vi "Parse Controls for xVDTs.vi"(2 "error in (no error)":errorcluster, 3 "Control Scalars":T2) -> (0 "error out":errorcluster, 1 "xVDTs":T1[](array[typedef]))   [LabVIEW 2011, in "Sensor Simulation Custom Device.lvlib"]
uses:
  Sensor Simulation Custom Device.lvlib
  <userlib>/_FPGA Interface Advanced Tools/FPGA Bitfile Utility/TypeDefs/Scalar Register Set.ctl
  <userlib>/_FPGA Interface Advanced Tools/FPGA Bitfile Utility/TypeDefs/Scalar Register.ctl
  TypeDefs/xVDT.ctl
  <vilib>/regexp/Match Regular Expression.xnode
  <userlib>/_FPGA Interface Advanced Tools/FPGA Bitfile Utility/FPGA Bitfile Utility.lvlib
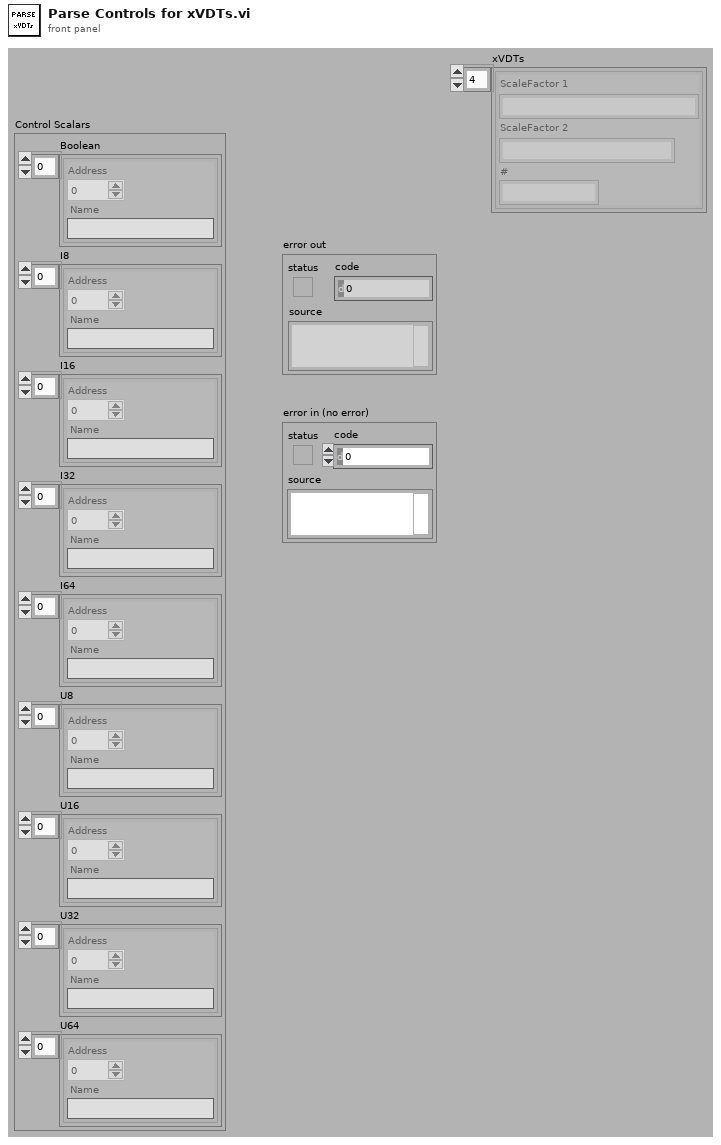
[diagram p1: front panel]
types:
  T1 = typedef "Sensor Simulation Custom Device.lvlib/xVDT.ctl" = cluster{"ScaleFactor 1":string, "ScaleFactor 2":string, "#":string}
  T2 = typedef "FPGA Bitfile Utility.lvlib/Scalar Register Set.ctl" = cluster{"Boolean":T3[], "I8":T3[], "I16":T3[], "I32":T3[], "I64":T3[], "U8":T3[], "U16":T3[], "U32":T3[], "U64":T3[]}
  T3 = typedef "FPGA Bitfile Utility.lvlib/Scalar Register.ctl" = cluster{"Address":u32, "Name":string}
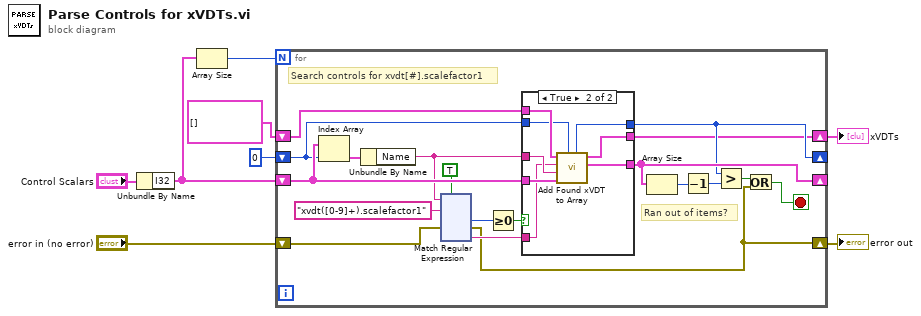
[diagram p0: block diagram]
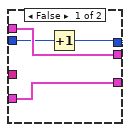
[diagram p2: hidden frame]
diagram:
  n1 = Unbundle By Name("Control Scalars") -> ("I32"=w3:T3[])
  n2 = Array Size(array=w3) -> (size(s)=w8:i32)
  n3 = for {
    N: w8 -> [_]
    shift-right: [w18] -> w4
    shift-left: T1[] [] -> [w26]
    shift-right: [w23] -> _
    shift-left: w3 -> [w25]
    shift-right: [w22] -> _
    shift-left: 0 -> [w17]
    shift-right: [w9] -> w1
    shift-left: "error in (no error)" -> [w11]
    stop <- w10 stop-if-true
    # "Search controls for xvdt[#].scalefactor1"
    # "Ran out of items?"
    n4 = Index Array(array=w25, index=w17) -> (element=w24:T3)
    n5 = Unbundle By Name(w24) -> ("Name"=w16:string)
    n6 = xnode "Match Regular Expression"("input string"=w16, "regular expression"="xvdt([0-9]+).scalefactor1", "error in"=w11, "ignore case? (F)"=TRUE) -> ("offset past match"=w13:i32, "error out"=w9:errorcluster, "submatch 1"=w12:string)  [unwired: 2 in, 3 out]
    n7 = Greater Or Equal To 0?(x=w13) -> (x >= 0?=w27:bool)
    n8 = case shown="True" w27 {
      tunnel: [w144 w152] -> w18
      tunnel: w26 -> [w144 w151]
      tunnel: w25 -> [w143 w150]
      tunnel: [w143 w149] -> w23
      tunnel: w17 -> [w142 w148]
      tunnel: [w141 w147] -> w22
      tunnel: w16 -> [_ w146]
      tunnel: w12 -> [_ w145]
      frame False {
        n9 = Increment(x=w142) -> (x+1=w141:i32)
      }
      frame True {
        n10 = call "Add Found xVDT to Array.vi"("Index Found"=w148, "Controls In"=w150, "ScaleFactor 1 Name"=w146, "xVDT Number"=w145, "xVDTs In"=w151) -> ("Controls Out"=w149:T3[], "xVDTs Out"=w152:T1[], "Next Index"=w147:i32)  [unwired: 4 in]
      }
    }
    n11 = Array Size(array=w23) -> (size(s)=w20:i32)
    n12 = Decrement(x=w20) -> (x-1=w19:i32)
    n13 = Greater?(x=w22, y=w19) -> (0:w21:bool)
    n14 = Or(x=w21, y=w9) -> (x .or. y?=w10:bool)
  }
  "xVDTs" <- w4
  "error out" <- w1
